vi "Robot Global Data.vi"() -> ()   [LabVIEW 2012]
doc: "This global VI can contain as many global variables as you need. Place a control on the panel, give it a good name. To read or write to it from a VI, drag the icon to the diagram of that VI. You can also drag from the project. Click on the node to change which global you access. You shouldn't have multiple locations writing to a global or it will cause a race-condition."
uses:
  <vilib>/Rock Robotics/WPI/Camera/WPI_CameraImageSize.ctl
  <vilib>/Rock Robotics/WPI/DriverStation/WPI_DriverStationRobotMode2.ctl
panel:
  in  "AutoStates":T1(ring)
  in  "BoxSpeed":T2
  in  "PickupState":T3(ring)
  in  "Actions":T4 {"Shooter" min=-1.0 max=1.0}
  in  "DIO":T5
  in  "Frisbee Count":i8 min=0 max=4 step=1
  in  "Robot Mode":T6
  out "Target Info":T7(array[cluster])
  in  "LED toggle rate (ms)":u32=20
  in  "image size":T8=enum."320x240"
  in  "Enable Vision":bool
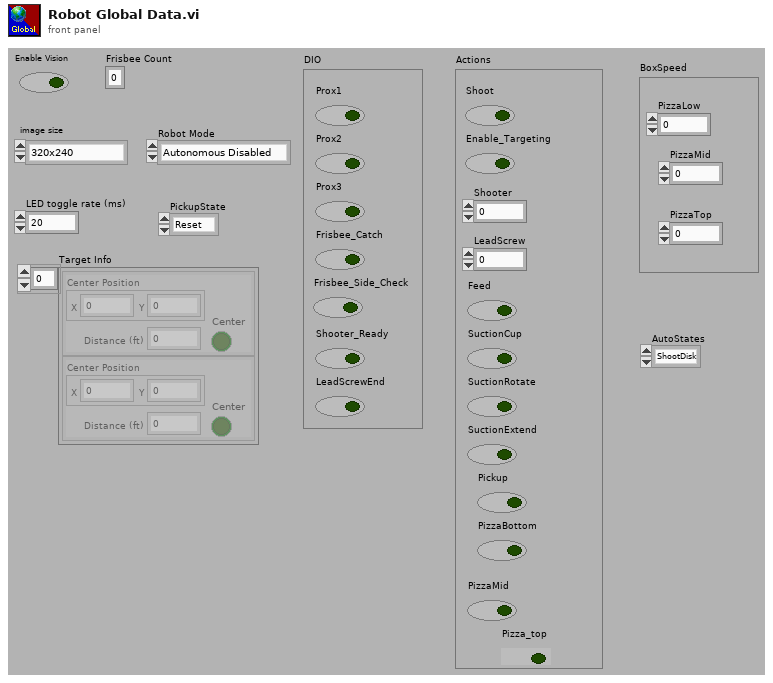
[diagram p1: front panel]
types:
  T1 = enum16{"ShootDisk", "AdvanceTwoDisk", "AdvanceOneDisk"}
  T2 = cluster{"PizzaLow":dbl, "PizzaMid":dbl, "PizzaTop":dbl}
  T3 = enum16{"Reset", "Ready", "Down", "Capture", "Lift", "Swing", "Release"}
  T4 = cluster{"Shoot":bool, "Enable_Targeting":bool, "Shooter":dbl, "LeadScrew":dbl, "Feed":bool, "SuctionCup":bool, "SuctionRotate":bool, "SuctionExtend":bool, "Pickup":bool, "PizzaBottom":bool, "PizzaMid":bool, "Pizza_top":bool}
  T5 = cluster{"Prox1":bool, "Prox2":bool, "Prox3":bool, "Frisbee_Catch":bool, "Frisbee_Side_Check":bool, "Shooter_Ready":bool, "LeadScrewEnd":bool}
  T6 = typedef "WPI_DriverStationRobotMode2.ctl" = enum16{"Autonomous Disabled", "Autonomous Enabled", "Teleop Disabled", "Teleop Enabled", "Timeout", "Finish", "Test Disabled", "Test Enabled"}
  T7 = cluster{"Center Position":cluster{"X":dbl, "Y":dbl}, "Distance (ft)":dbl, "Center":bool}[]
  T8 = typedef "WPI_CameraImageSize.ctl" = enum16{"640x480", "320x240", "160x120"}
diagram:
